vi "save_setup.vi"(8 "error in (no error)":errorcluster, 9 "Setup # (0-9)":u8, 10 "Channel":string="1", 11 "VISA Refnum in":refnum<visa-resource-name>) -> (0 "error out":errorcluster, 3 "VISA Refnum out":refnum<visa-resource-name>)   [LabVIEW 2018, in "Aim-TTi CPX400SP.lvlib"]
uses:
  <instrlib>/Aim-TTi CPX400SP/Aim-TTi CPX400SP.lvlib
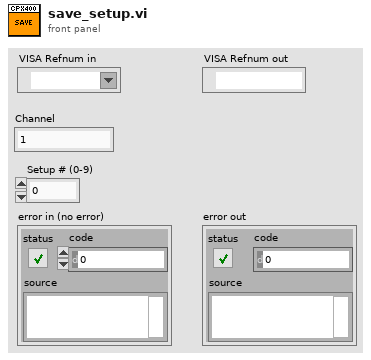
[diagram p1: front panel]
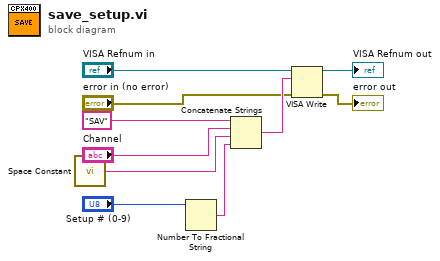
[diagram p0: block diagram]
diagram:
  n1 = call <vilib>:"Space Constant.vi"() -> ("String"=w3:string)
  n2 = Number To Fractional String(number="Setup # (0-9)") -> (F-format string=w1:string)  [unwired: 3 in]
  n3 = Concatenate Strings("SAV" ("string"), "Channel", w3, w1) -> (w8:string)
  n4 = VISA Write(VISA resource name="VISA Refnum in", write buffer=w8, error in (no error)="error in (no error)") -> (VISA resource name out=→"VISA Refnum out":refnum<visa-resource-name>, error out=→"error out":errorcluster)  [unwired: 1 out]
